vi "FromClusterToTagBusScript.vi"(5 "process":T1, 7 "output":T2, 8 "error in":errorcluster, 10 "input":T3, 11 "runtime class path":path) -> (0 "error out":errorcluster)   [LabVIEW 2013]
doc: "THis Vi scripts the index cluster and the VI to convert from a cluster into Tagbus"
uses:
  Controls/input script control.ctl
  Controls/output script control.ctl
  Controls/processing script control.ctl
  Controls/ControlsProperties.ctl
  <vilib>/Utility/miscctls.llb/LVPointTypeDef.ctl
  Controls/StateCluster.ctl
  Controls/initialized references.ctl
  Controls/interface VI type.ctl
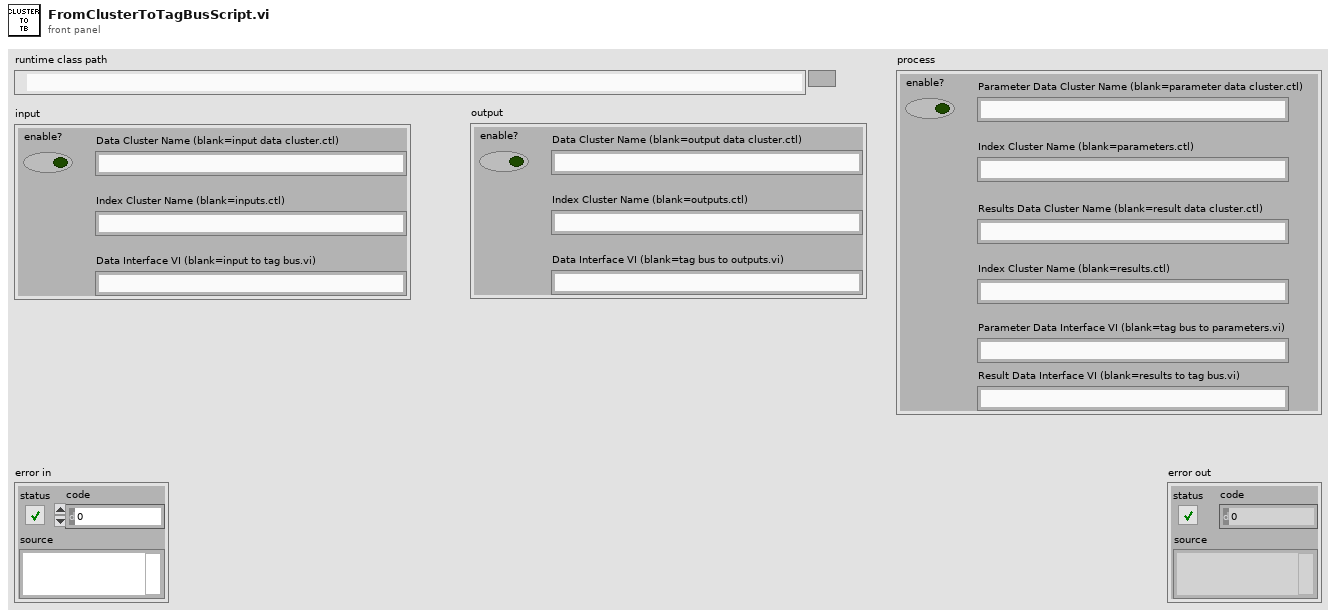
[diagram p1: front panel]
types:
  T1 = typedef "processing script control.ctl" = cluster{"enable?":bool, "Parameter Data Cluster Name (blank=parameter data cluster.ctl)":string, "Index Cluster Name (blank=parameters.ctl)":string, "Results Data Cluster Name (blank=result data cluster.ctl)":string, "Index Cluster Name (blank=results.ctl)":string, "Parameter Data Interface VI (blank=tag bus to parameters.vi)":string, "Result Data Interface VI (blank=results to tag bus.vi)":string}
  T2 = typedef "output script control.ctl" = cluster{"enable?":bool, "Data Cluster Name (blank=output data cluster.ctl)":string, "Index Cluster Name (blank=outputs.ctl)":string, "Data Interface VI (blank=tag bus to outputs.vi)":string}
  T3 = typedef "input script control.ctl" = cluster{"enable?":bool, "Data Cluster Name (blank=input data cluster.ctl)":string, "Index Cluster Name (blank=inputs.ctl)":string, "Data Interface VI (blank=input to tag bus.vi)":string}
  T4 = typedef "ControlsProperties.ctl" = cluster{"label":string, "terminal index":u32, "indicator":bool, "location":T5}
  T5 = typedef "LVPointTypeDef.ctl" = cluster{"Horizontal":i16, "Vertical":i16}
  T6 = typedef "initialized references.ctl" = cluster{"data ctl":refnum<vi>, "index ctl":refnum<vi>, "interface vi":refnum<vi>, "vi type":T7}
  T7 = typedef "interface VI type.ctl" = enum16{"tb to data", "data to tb"}
  T8 = typedef "StateCluster.ctl" = cluster{"base cluster":variant, "vi refs":T6}
  T9 = typedef "TerminalReferences.ctl" = cluster{"Cluster":refnum<vi>, "Index Cluster":refnum<vi>, "tag bus in":refnum<vi>, "tag bus out":refnum<vi>, "error in ":refnum<vi>, "error out":refnum<vi>}
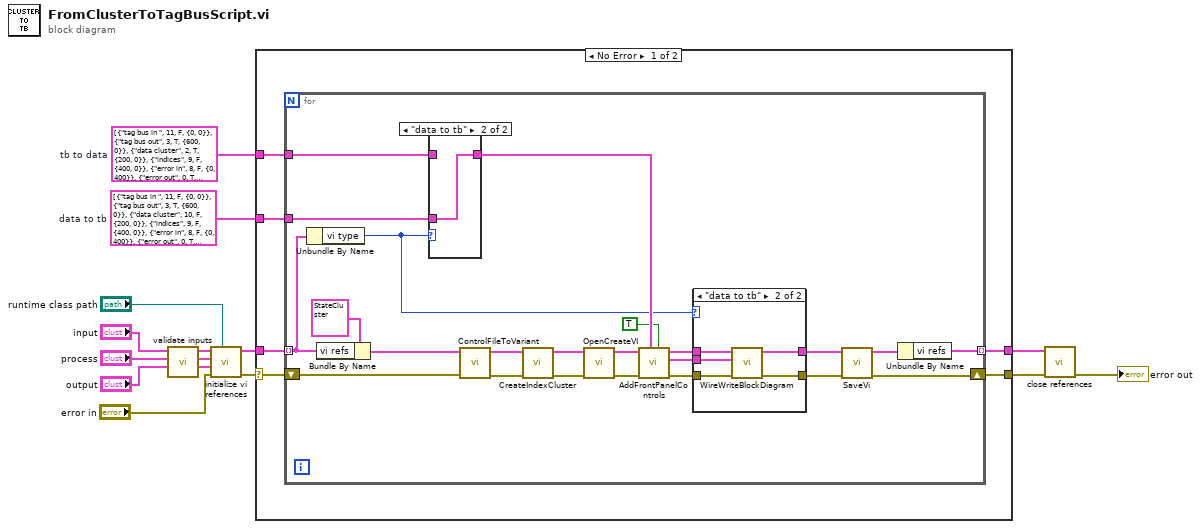
[diagram p0: block diagram]
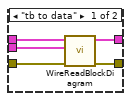
[diagram p2: hidden frame]
diagram:
  w1 = T4[] [{"label"="tag bus in ", "terminal index"=11, "indicator"=FALSE, "location"={"Horizontal"=0, "Vertical"=0}}, {"label"="tag bus out", "terminal index"=3, "indicator"=TRUE, "location"={"Horizontal"=600, "Vertical"=0}}, {"label"="data cluster", "terminal index"=10, "indicator"=FALSE, "location"={"Horizontal"=200, "Vertical"=0}}, {"label"="indices", "terminal index"=9, "indicator"=FALSE, "location"={"Horizontal"=400, "Vertical"=0}}, {"label"="error in", "terminal index"=8, "indicator"=FALSE, "location"={"Horizontal"=0, "Vertical"=400}}, {"label"="error out", "terminal index"=0, "indicator"=TRUE, "location"={"Horizontal"=600, "Vertical"=400}}]  # data to tb
  w2 = T4[] [{"label"="tag bus in ", "terminal index"=11, "indicator"=FALSE, "location"={"Horizontal"=0, "Vertical"=0}}, {"label"="tag bus out", "terminal index"=3, "indicator"=TRUE, "location"={"Horizontal"=600, "Vertical"=0}}, {"label"="data cluster", "terminal index"=2, "indicator"=TRUE, "location"={"Horizontal"=200, "Vertical"=0}}, {"label"="indices", "terminal index"=9, "indicator"=FALSE, "location"={"Horizontal"=400, "Vertical"=0}}, {"label"="error in", "terminal index"=8, "indicator"=FALSE, "location"={"Horizontal"=0, "Vertical"=400}}, {"label"="error out", "terminal index"=0, "indicator"=TRUE, "location"={"Horizontal"=600, "Vertical"=400}}]  # tb to data
  n1 = call "validate inputs.vi"("output in"="output", "process in"="process", "input in"="input") -> ("output out"=w10:T2, "process out"=w11:T1, "input out"=w12:T3)  [unwired: 6 in]
  n2 = call "initialize vi references.vi"("runtime class path"="runtime class path", "error in"="error in", "output in"=w10, "process in"=w11, "input in"=w12) -> ("error out"=w8:errorcluster, "initialized references"=w7:T6[])  [unwired: 5 in]
  n3 = case shown="No Error" w8 {
    selector: w8 -> [w20 w58]
    tunnel: w7 -> [w21 w57]
    tunnel: [w19 w58] -> w4
    tunnel: [w16 w57] -> w5
    tunnel: w2 -> [w18 _]
    tunnel: w1 -> [w17 _]
    frame No Error {
      n4 = for {
        tunnel: w21 -> [w41] mode=indexing
        shift-right: [w24] -> w19
        shift-left: w20 -> [w39]
        tunnel: w18 -> [w44]
        tunnel: w17 -> [w43]
        tunnel: [w22] -> w16 mode=indexing
        n5 = Unbundle By Name(w41) -> ("vi type"=w30:T7)
        n6 = Bundle By Name(cluster=T8 {"base cluster"=variant, "vi refs"={"data ctl"=refnum, "index ctl"=refnum, "interface vi"=refnum, "vi type"=enum."tb to data"}} ("State"), "vi refs"=w41) -> (w40:T8)
        n7 = case shown="\"data to tb\"" w30 {
          tunnel: [w55 w56] -> w32
          tunnel: w44 -> [w55 _]
          tunnel: w43 -> [_ w56]
          frame "tb to data" {
          }
          frame "data to tb" {
          }
        }
        n8 = call "ControlFileToVariant.vi"("error in"=w39, "State"=w40) -> ("error out"=w37:errorcluster, "State out"=w38:T8)  [unwired: 8 in]
        n9 = call "CreateIndexCluster.vi"("error in"=w37, "State"=w38) -> ("error out"=w35:errorcluster, "State out"=w36:T8)  [unwired: 8 in]
        n10 = call "OpenCreateVI.vi"("error in"=w35, "State"=w36) -> ("error out"=w34:errorcluster, "State out"=w33:T8)  [unwired: 8 in]
        n11 = call "AddFrontPanelControls.vi"("Open Front Panel"=TRUE, "Control Properties"=w32, "error in"=w34, "State"=w33) -> ("error out"=w27:errorcluster, "Terminal References"=w28:T9, "State out"=w29:T8)  [unwired: 5 in]
        n12 = case shown="\"data to tb\"" w30 {
          tunnel: w29 -> [w49 w54]
          tunnel: w28 -> [w48 w53]
          tunnel: w27 -> [w47 w52]
          tunnel: [w46 w51] -> w25
          tunnel: [w45 w50] -> w26
          frame "tb to data" {
            n13 = call "WireReadBlockDiagram.vi"("error in"=w47, "Terminal References"=w48, "State"=w49) -> ("error out"=w46:errorcluster, "State out"=w45:T8)  [unwired: 7 in]
          }
          frame "data to tb" {
            n14 = call "WireWriteBlockDiagram.vi"("error in"=w52, "Terminal References"=w53, "State"=w54) -> ("error out"=w51:errorcluster, "State out"=w50:T8)  [unwired: 7 in]
          }
        }
        n15 = call "SaveVi.vi"("error in"=w25, "State"=w26) -> ("error out"=w24:errorcluster, "State out"=w23:T8)  [unwired: 8 in]
        n16 = Unbundle By Name(w23) -> ("vi refs"=w22:T6)
      }
    }
    frame Error {
    }
  }
  n17 = call "close references.vi"("error in"=w4, "initialized references"=w5) -> ("error out"=→"error out":errorcluster)  [unwired: 9 in]
